vi "API_DB.AddReticleInDB.vi"(0 "Database in":refnum<class "Database.lvclass">, 1 "Wait (F)":bool, 2 "InventoryRecord.Location.Module":u16, 5 "Table":string, 7 "InventoryRecord.Stocker":T1 items=["Main", "Exp1", "Exp2"], 9 "InventoryRecord.ReticleID":string, 11 "error in (no error)":errorcluster, 12 "Timeout (ms)":u32, 13 "InventoryRecord.Location.Row":u16, 14 "InventoryRecord.Location.Column":u16) -> (4 "Database out":refnum<class "Database.lvclass">, 6 "Slot":string, 15 "error out":errorcluster)   [LabVIEW 2022 SP3]
doc: "Developed by Kevin Thompson\nkevin@thompsonengineering.net\n\nCopyright 2018\nThompson Engineering, LLC"
uses:
  Database.lvclass
  DataTypes/AsynCmd_Temp01--enum.ctl
  DataTypes/GenericQuery--Cluster.ctl
  DataTypes/SQLQuery--Enum.ctl
  Database.lvclass/Database.ctl
  DataTypes/Stocker--Enum.ctl
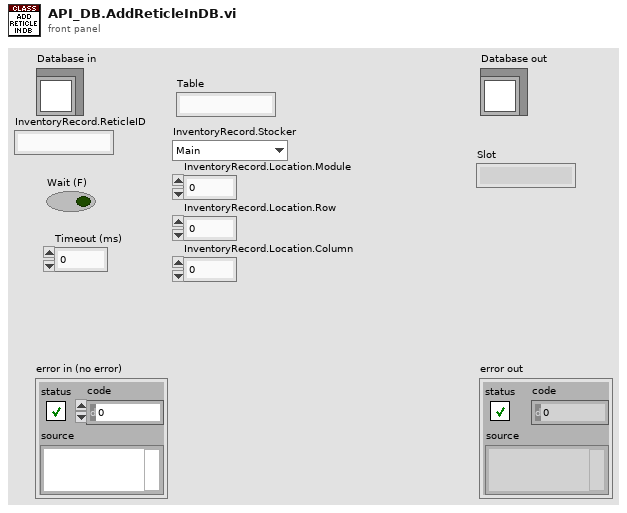
[diagram p1: front panel]
types:
  T1 = typedef "Stocker--Enum.ctl" = u16
  T2 = typedef "SQLQuery--Enum.ctl" = enum16{"GetAllMaterials", "GetAllColors"}
  T3 = typedef "GenericQuery--Cluster.ctl" = cluster{"Query":T2, "Table":string}
  T4 = typedef "Database.lvclass/AsynCmd_Temp01--enum.ctl" = enum16{"DB.DeleteRecord", "DB.UpdateRecord", "DB.InsertRecord", "DB.SelectRecord", "DB.ExecuteSQLCommand", "DB.FindFirstSlot", "DB.GenericSQLQuery"}
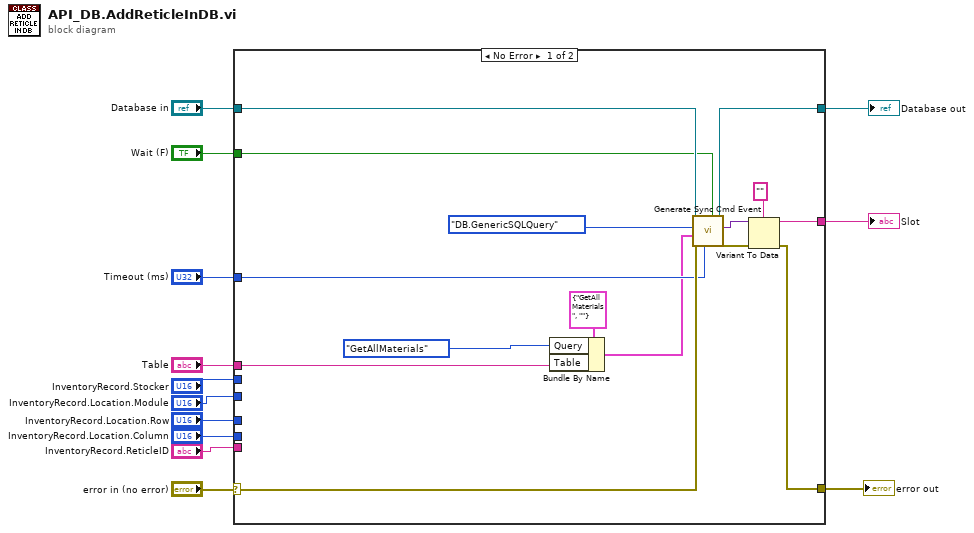
[diagram p0: block diagram]
diagram:
  n1 = case shown="No Error" "error in (no error)" {
    selector: "error in (no error)" -> [w26 w30]
    tunnel: [w21 w30] -> w12
    tunnel: [w27 w29] -> w10
    tunnel: "Database in" -> [w28 w29]
    tunnel: [w23 _] -> w7
    tunnel: "Wait (F)" -> [w20 _]
    tunnel: "Timeout (ms)" -> [w19 _]
    tunnel: "Table" -> [w14 _]
    tunnel: "InventoryRecord.Stocker" -> [_ _]
    tunnel: "InventoryRecord.Location.Module" -> [_ _]
    tunnel: "InventoryRecord.Location.Row" -> [_ _]
    tunnel: "InventoryRecord.Location.Column" -> [_ _]
    tunnel: "InventoryRecord.ReticleID" -> [_ _]
    frame No Error {
      n2 = Bundle By Name(cluster=T3 {"Query"=enum."GetAllMaterials", "Table"=""}, "Query"=SQLQuery--Enum."GetAllMaterials", "Table"=w14) -> (w15:T3)
      n3 = call "Generate Sync Cmd Event.vi"("Wait (F)"=w20, "Timeout (ms)"=w19, "error in (no error)"=w26, "vData"=w15, "AsyncCmd"=AsynCmd_Temp01--enum."DB.GenericSQLQuery", "Database in"=w28) -> ("error out"=w22:errorcluster, "Return Value"=w24:variant, "Database out"=w27:refnum<class "Database.lvclass">)  [unwired: 3 in]
      n4 = Variant To Data(error in=w22, type="", Variant=w24) -> (data=w23:string, error out=w21:errorcluster)
    }
    frame Error {
    }
  }
  "error out" <- w12
  "Database out" <- w10
  "Slot" <- w7
